vi "ADAM6018.vi"(4 "Scan Period":dbl format="%.2f", 5 "Previous Scan Value":dbl format="%.2f", 6 "Present scan array":dbl[](array[numeric]) format="%.2f", 7 "Value to Output":dbl format="%.2f", 8 "Ch Description":T1={"Ch Name"="", "Type"="", "Function"=enum."Analogue Input", "Ch State"=enum."On", "Calibration type"="", "A"=0.0, "B"=0.0, "C"=0.0, "D"=0.0, "Comments"="", "Address"={"Main"=0, "Ch."=0, "Sub"=0, "Port Name"="192.168.120.110"}, "String"="", "Duty"=65535} {"Duty" format="%016b"; "D" format="%#_5g"; "C" format="%#_5g"; "B" format="%#_5g"; "A" format="%#_5g"}, 9 "Ch names":string[](array[string])) -> (0 "Scan comment":string, 1 "Output":dbl format="%.3f")   [LabVIEW 2016]
uses:
  ADAM Client/Sub VIs/ADAM Controls/Ch_description_ADAM.ctl
  ADAM Client/Sub VIs/ADAM Controls/Module_type_ADAM.ctl
  ADAM Client/Sub VIs/ADAM Controls/Function_ADAM.ctl
  ADAM Client/Sub VIs/ADAM Controls/Channel_State.ctl
  ADAM Client/Sub VIs/ADAM Controls/Calib_type_ADAM.ctl
  ADAM Client/Sub VIs/ADAM Controls/Address.ctl
  ADAM Serial/Serial Link Layer/NI_Modbus_Cleaned/NI Modbus121Clean.llb/MB Modbus Command.ctl
  <vilib>/Utility/error.llb/DialogType.ctl
panel:
  out "Port Name":string="192.168.120.110"
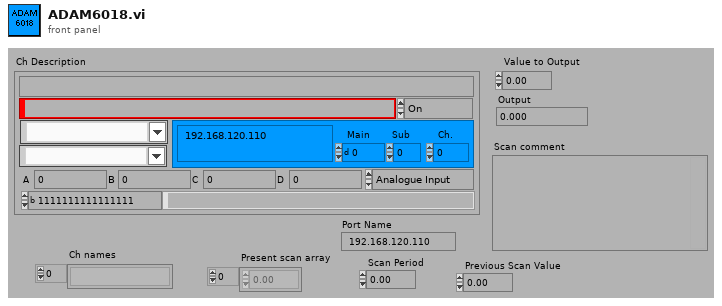
[diagram p1: front panel]
types:
  T1 = typedef "Ch_description_ADAM.ctl" = cluster{"Ch Name":string, "Type":T2, "Function":T3, "Ch State":T4, "Calibration type":T5, "A":dbl, "B":dbl, "C":dbl, "D":dbl, "Comments":string, "Address":T6, "String":string, "Duty":u16}
  T2 = typedef "Module_type_ADAM.ctl" = string
  T3 = typedef "Function_ADAM.ctl" = enum16{"Analogue Input", "Digital Input", "Event counter", "Event rate", "Analogue Output", "Digital Output", "Relay Output"}
  T4 = typedef "Channel_State.ctl" = enum16{"On", "Off", "Always On", "Always Off"}
  T5 = typedef "Calib_type_ADAM.ctl" = string
  T6 = typedef "Address.ctl" = cluster{"Main":i32, "Ch.":i32, "Sub":i32, "Port Name":string}
  T7 = typedef "DialogType.ctl" = u16
  T8 = typedef "MB Modbus Command.ctl" = cluster{"Function Code":u8, "Starting Address":u16, "Quantity":u16, "Data":u16[], "Discrete":bool[]}
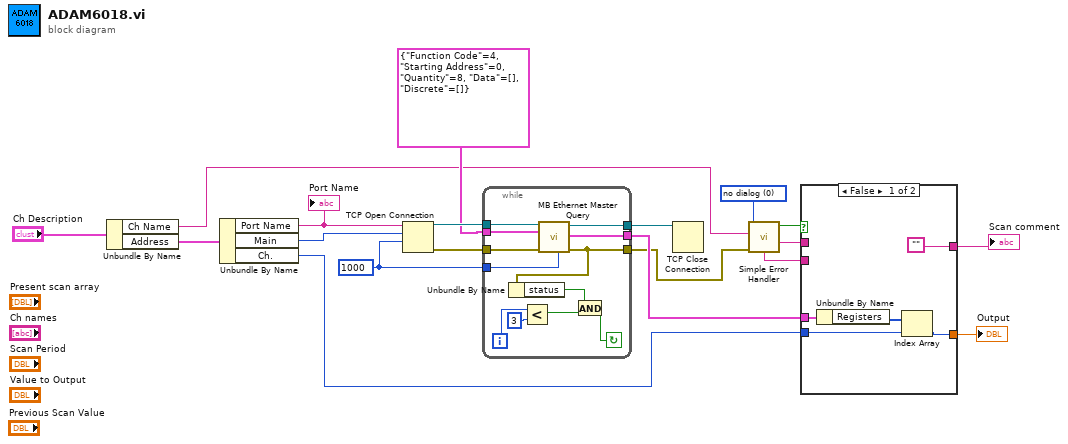
[diagram p0: block diagram]
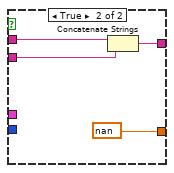
[diagram p2: hidden frame]
diagram:
  w14 = T7 0 items=["no dialog", "OK message", "continue or stop message", "OK message + warnings", "continue/stop + warnings"] ("type of dialog (OK msg:1)")
  w12 = 1000 ("Timeout")
  n1 = Unbundle By Name("Ch Description") -> ("Ch Name"=w5:string, "Address"=w7:T6)
  n2 = Unbundle By Name(w7) -> ("Port Name"=w9:string, "Main"=w8:i32, "Ch."=w6:i32)
  "Port Name" <- w9
  n3 = TCP Open Connection(address=w9, remote port or service name=w8, timeout ms (60000)=w12) -> (connection ID=w18:refnum<k5>, error out=w19:errorcluster)  [unwired: 1 in, 1 out]
  n4 = while {
    tunnel: w19 -> [w31]
    tunnel: T8 {"Function Code"=4, "Starting Address"=0, "Quantity"=8, "Data"=[], "Discrete"=[]} ("Modbus Command") -> [w29]
    tunnel: [w27] -> w16
    tunnel: w12 -> [w26]
    tunnel: [w25] -> w1
    tunnel: w18 -> [w30]
    tunnel: [w28] -> w17
    i -> [w23]
    stop <- w24 continue-if-true
    n5 = Less?(x=w23, y=3) -> (x < y?=w21:bool)
    n6 = call "MB Ethernet Master Query.vi"("Timeout"=w26, "error in (no error)"=w31, "Modbus Command"=w29, "TCP Connection Refnum in"=w30) -> ("error out"=w25:errorcluster, "Registers"=w27:cluster{"Registers":u16[], "Discrete":bool[]}, "TCP Connection Refnum (dup)"=w28:refnum<k5>)  [unwired: 3 in, 2 out]
    n7 = Unbundle By Name(w25) -> ("status"=w20:bool)
    n8 = And(x=w20, y=w21) -> (x .and. y?=w24:bool)
  }
  n9 = TCP Close Connection(connection ID=w17) -> ()  [unwired: 1 in, 3 out]
  n10 = call <vilib>:"Simple Error Handler.vi"("error source (\" \")"=w5, "type of dialog (OK msg:1)"=w14, "error in (no error)"=w1) -> ("error?"=w4:bool, "source out"=w11:string, "message"=w13:string)  [unwired: 4 out]
  n11 = case shown="False" w4 {
    tunnel: w16 -> [w36 _]
    tunnel: w13 -> [_ w38]
    tunnel: w11 -> [_ w39]
    tunnel: w6 -> [w34 _]
    tunnel: ["" w37] -> w3
    tunnel: [w33 nan ("t")] -> w2
    frame False {
      n12 = Unbundle By Name(w36) -> ("Registers"=w35:u16[])
      n13 = Index Array(array=w35, index=w34) -> (element=w33:u16)
    }
    frame True {
      n14 = Concatenate Strings(w39, w38) -> (w37:string)
    }
  }
  "Output" <- w2
  "Scan comment" <- w3
